vi "Read Common Parameters.vi"(8 "error in (no error)":errorcluster, 11 "Schedule Block in":refnum<class "Schedule Block.lvclass">) -> (0 "error out":errorcluster, 2 "Common Parameters":string[][](array[string]), 3 "Schedule Block out":refnum<class "Schedule Block.lvclass">)   [LabVIEW 2020, in "Run Utilities.lvlib" / "Schedule Block.lvclass"]
uses:
  Schedule Block.lvclass
  Schedule Block.lvclass/Schedule Block.ctl
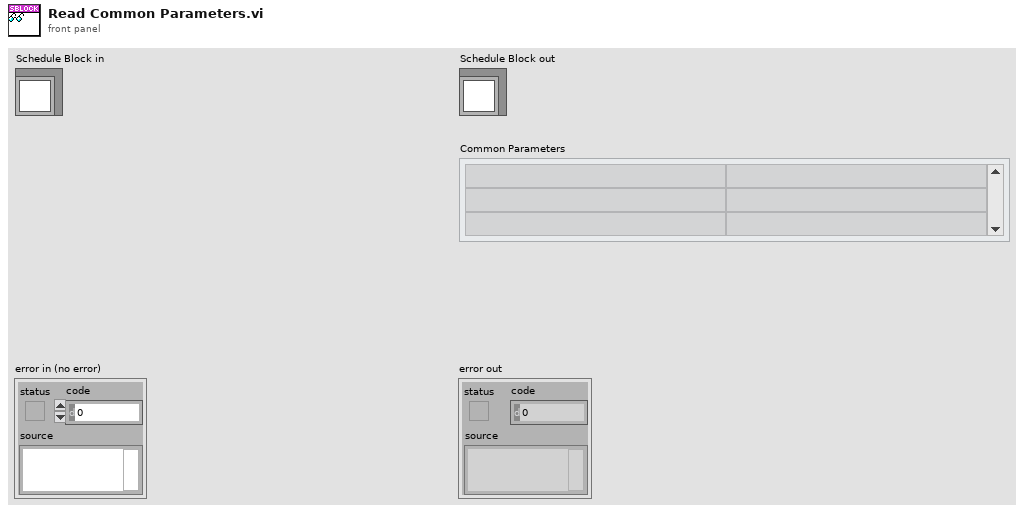
[diagram p1: front panel]
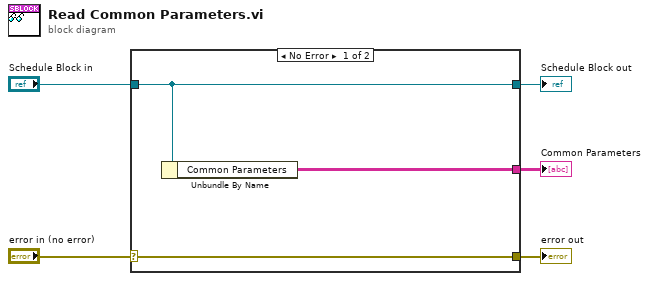
[diagram p0: block diagram]
diagram:
  n1 = case shown="No Error" "error in (no error)" {
    selector: "error in (no error)" -> [w8 w9]
    tunnel: [w8 w9] -> w4
    tunnel: [w7 w10] -> w2
    tunnel: "Schedule Block in" -> [w7 w10]
    tunnel: [w6 _] -> w1
    frame No Error {
      n2 = Unbundle By Name(w7) -> ("Common Parameters"=w6:string[][])
    }
    frame Error {
    }
  }
  "error out" <- w4
  "Schedule Block out" <- w2
  "Common Parameters" <- w1
